vi "Disconnect OPC UA.vi"(8 "error in (no error)":errorcluster, 10 "FGV Name":string="Ignition Ref", 11 "subscription IDs":T1[](array[typedef])) -> (0 "error out":errorcluster)   [LabVIEW 2021, in "OPCUA.lvlib"]
uses:
  <vilib>/OPCUA/controls/Subscription ID.ctl
  <vilib>/OPCUA/controls/OPC UA Client Refnum.ctl
  OPCUA.lvlib
  <vilib>/OPCUA/NI OPC UA Client.lvlib
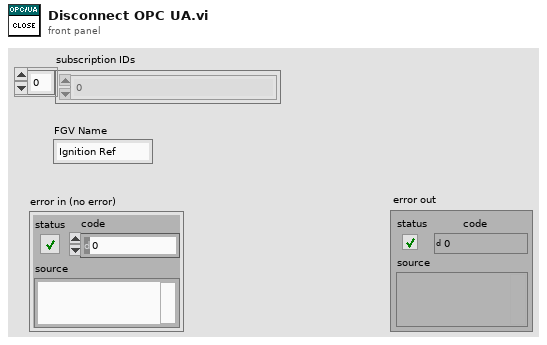
[diagram p1: front panel]
types:
  T1 = typedef "Subscription ID.ctl" = u32
  T2 = typedef "OPC UA Client Refnum.ctl" = refnum<k21>
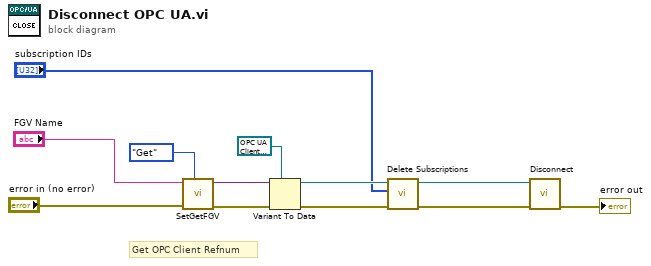
[diagram p0: block diagram]
diagram:
  # "Get OPC Client Refnum"
  n1 = call "SetGetFGV.vi"("Method (Get)"=enum16{"Get", "Set"}."Get", "error in"="error in (no error)", "FGVname"="FGV Name") -> ("error out"=w3:errorcluster, "Data out"=w5:variant)  [unwired: 7 in]
  n2 = Variant To Data(error in=w3, type=T2 refnum ("OPC UA client refnum out"), Variant=w5) -> (data=w4:T2, error out=w2:errorcluster)
  n3 = call <vilib>:"Delete Subscriptions.vi"("error in (no error)"=w2, "subscription IDs"="subscription IDs", "OPC UA client refnum in"=w4) -> ("error out"=w12:errorcluster, "OPC UA client refnum out"=w10:T2)  [unwired: 6 in, 1 out]
  n4 = call <vilib>:"Disconnect.vi"("error in (no error)"=w12, "OPC UA client refnum in"=w10) -> ("error out"=→"error out":errorcluster)  [unwired: 9 in]
